vi "Fetch.vi"   [LabVIEW 2011, in "Tektronix 7000 Series.lvlib"]
doc: "Returns the waveform that an oscilloscope acquires for a channel you specify. An acquisition that you initiate before calling this VI generates the waveform."
uses:
  Tektronix 7000 Series.lvlib
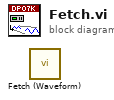
[diagram p0: block diagram]
diagram:
  n1 = call "Fetch (Waveform).vi"() -> ()  [unwired: 9 in, 3 out]
